vi "AMC Send Network Message.vi"(1 "Priority Message (F)":bool, 4 "Message Attributes":T1, 5 "Receiver Host":string, 6 "Acknowledge Message (F)":bool, 7 "Receiver Process":string, 8 "error in (no error)":errorcluster, 9 "Message Value":string, 10 "Message Name":string, 11 "Message Queue in":T2) -> (0 "error out":errorcluster, 3 "Message Queue out":T2)   [LabVIEW 2017]
doc: "This VI adds a message to the local message queue provided by the queue reference or to another message queue on the local target based on the receiver process name."
uses:
  subVIs/TypeDefs/amc_Message.ctl
  Tools/Keyed Array/Tools_KeyedArray KeyedArray.ctl
  subVIs/TypeDefs/amc_Message Queue.ctl
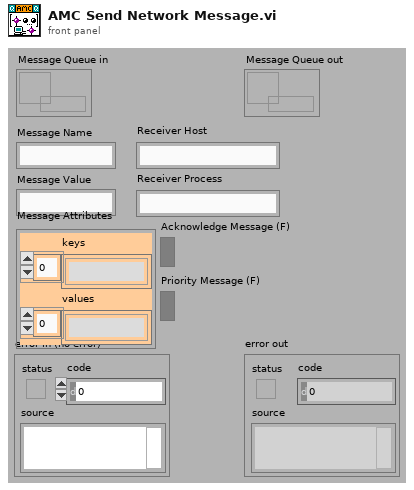
[diagram p1: front panel]
types:
  T1 = typedef "Tools_KeyedArray KeyedArray.ctl" = cluster{"keys":string[], "values":string[]}
  T2 = typedef "amc_Message Queue.ctl" = refnum<queue>
  T3 = typedef "amc_Message.ctl" = cluster{"Name":string, "Value":string, "Attributes":T1, "Receiver Host":string, "Receiver Process":string, "Source Host":string, "Source Process":string, "Priority Message":bool, "Acknowledge Message":bool}
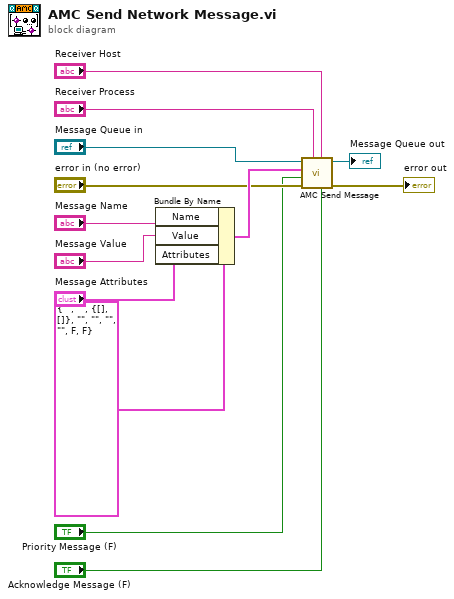
[diagram p0: block diagram]
diagram:
  n1 = Bundle By Name(cluster=T3 {"Name"="", "Value"="", "Attributes"={"keys"=[], "values"=[]}, "Receiver Host"="", "Receiver Process"="", "Source Host"="", "Source Process"="", "Priority Message"=FALSE, "Acknowledge Message"=FALSE} ("Message"), "Name"="Message Name", "Value"="Message Value", "Attributes"="Message Attributes") -> (w13:T3)
  n2 = call "AMC Send Message.vi"("Acknowledge Message (F)"="Acknowledge Message (F)", "Receiver Host"="Receiver Host", "Receiver Process"="Receiver Process", "error in (no error)"="error in (no error)", "Priority Message (F)"="Priority Message (F)", "Message"=w13, "Message Queue in"="Message Queue in") -> ("error out"=→"error out":errorcluster, "Message Queue out"=→"Message Queue out":T2)  [unwired: 1 in, 2 out]
